vi "TrackerColor.vi"() -> ()   [LabVIEW 2015]
panel:
  in  "Example Image Path":path
  out "Image Out 2":T1(plugin-control)
  in  "Color":u32(colorbox)=16711680
  out "Image Out":T1(plugin-control)
  out "Image":T1(plugin-control)
  in  "Stop":bool
  out "Progress Bar":i32(slide) max=115 scale=1.0..115.0
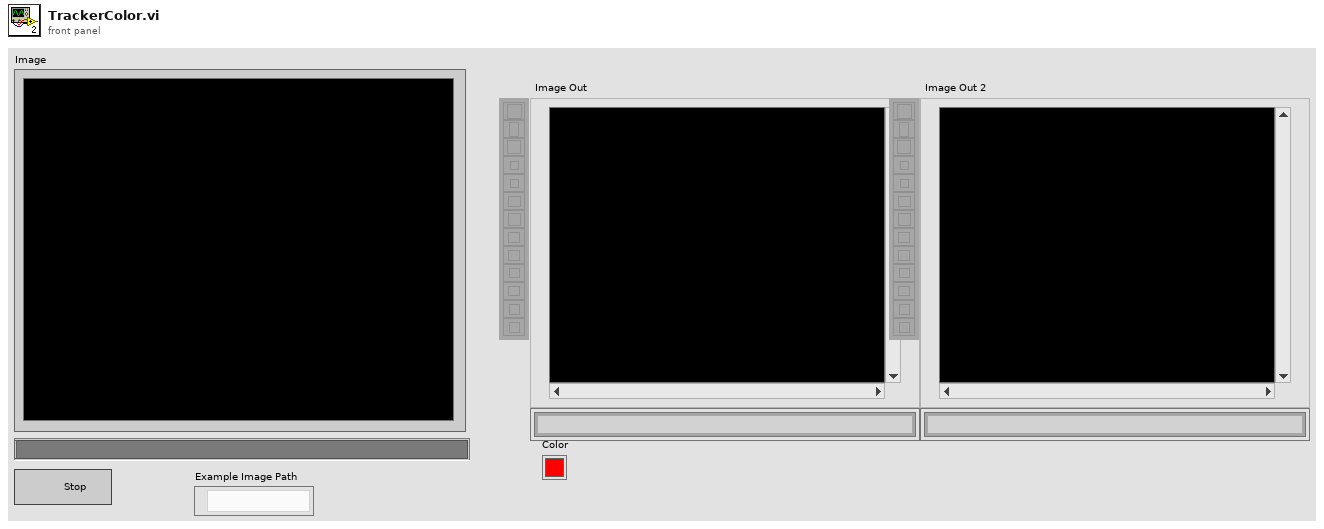
[diagram p1: front panel]
types:
  T1 = typedef "IMAQ Image.ctl" = refnum<image>
  T2 = typedef "IMAQ AVI2 Refnum.ctl" = refnum<k20>
  T3 = typedef "Image Type" = u32
  T4 = cluster{"Width":u32, "Height":u32, "Frames Per Second":u32, "Codec":string, "Has Data":bool}
  T5 = cluster{"Position":cluster{"x":sgl, "y":sgl}, "Angle":sgl, "Scale":sgl, "Score":sgl, "Bounding Box":cluster{"x":sgl, "y":sgl}[]}[]
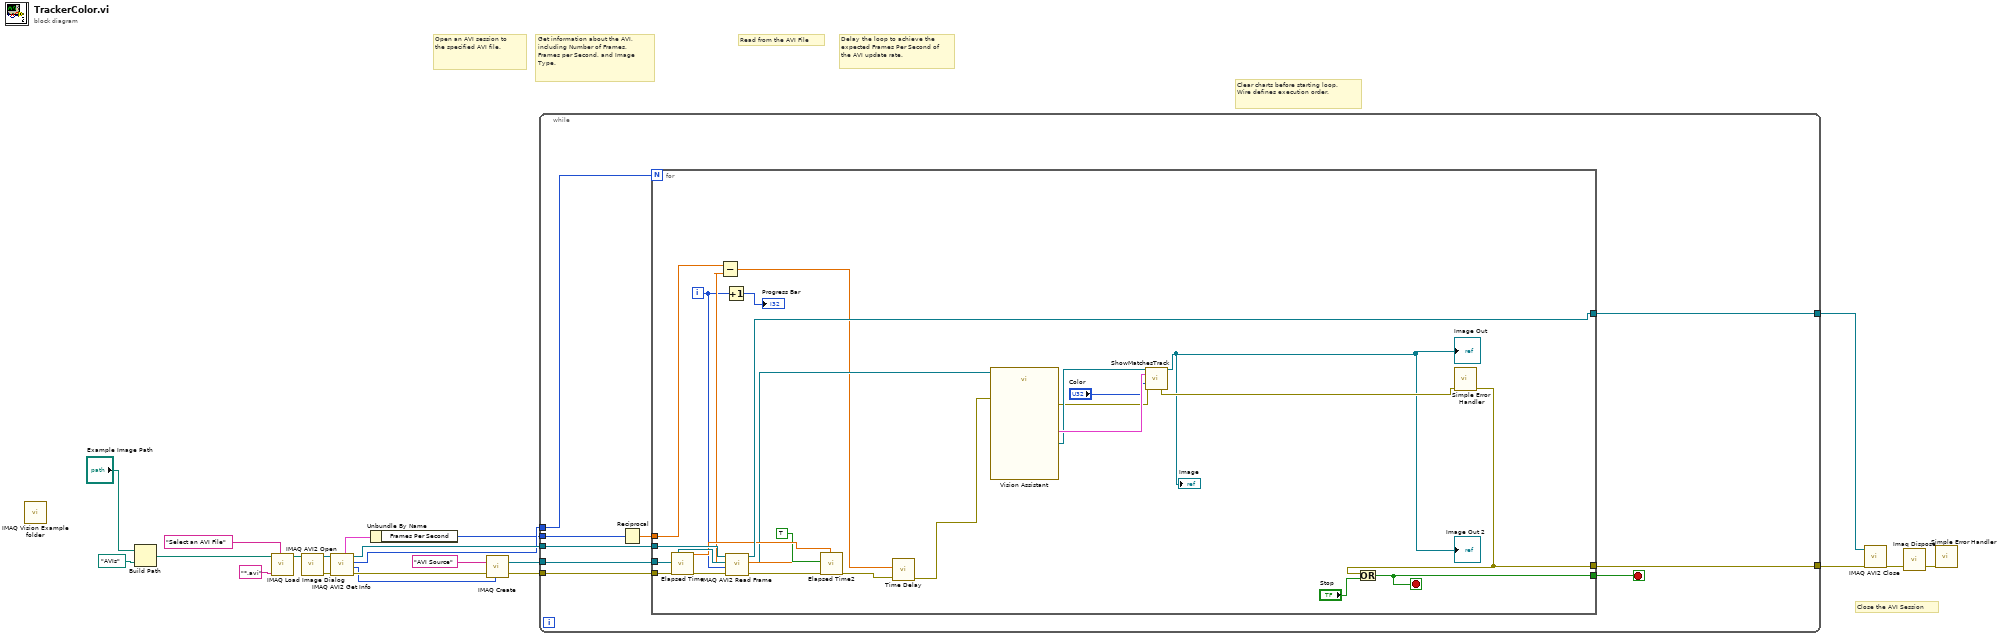
[diagram p0: block diagram]
diagram:
  # "Close the AVI Session"
  # "Clear charts before starting loop. Wire defines execution order."
  # "Read from the AVI File"
  # "Get information about the AVI, including Number of Frames, Frames per Second, and Image Type."
  # "Open an AVI session to the specified AVI file."
  # "Delay the loop to achieve the expected Frames Per Second of the AVI update rate."
  n1 = call "IMAQ Vision Example folder.vi"() -> ()  [unwired: 11 in, 1 out]
  n2 = Build Path(base path="Example Image Path", name or relative path=path "AVIs") -> (appended path=w6:path)
  n3 = call "IMAQ Load Image Dialog"("Prompt"="Select an AVI File" ("prompt"), "Pattern"="*.avi", "Start Path"=w6) -> ("Path"=w5:path)  [unwired: 6 in, 2 out]
  n4 = call "IMAQ AVI2 Open"("AVI File Path"=w5) -> ("error out"=w18:errorcluster, "AVI Refnum"=w17:T2)  [unwired: 2 in, 7 out]
  n5 = call "IMAQ AVI2 Get Info"("error in (no error)"=w18, "AVI Refnum"=w17) -> ("error out"=w14:errorcluster, "Image Type"=w9:T3, "Number of Frames"=w3:u32, "AVI Refnum (duplicate)"=w11:T2, "Frame Data"=w19:T4)  [unwired: 5 out]
  n6 = Unbundle By Name(w19) -> ("Frames Per Second"=w2:u32)
  n7 = call "IMAQ Create"("Image Name"="AVI Source", "Image Type"=w9, "error in (no error)"=w14) -> ("New Image"=w12:T1, "error out"=w13:errorcluster)  [unwired: 1 in, 1 out]
  n8 = while {
    tunnel: [w30] -> w16
    tunnel: [w29] -> w15
    tunnel: w13 -> [w28]
    tunnel: w12 -> [w27]
    tunnel: w11 -> [w26]
    tunnel: w2 -> [w25]
    tunnel: w3 -> [w23]
    stop <- w22 stop-if-true
    n9 = Reciprocal(x=w25) -> (1/x=w24:dbl)
    n10 = for {
      N: w23 -> [_]
      tunnel: w27 -> [w54]
      tunnel: [w53] -> w29
      tunnel: [w38] -> w30
      tunnel: w28 -> [w52]
      tunnel: w26 -> [w55]
      tunnel: w24 -> [w50]
      tunnel: [w40] -> w22
      i -> [w43]
      stop <- w40 stop-if-true
      n11 = call "Elapsed Time"("error in (no error)"=w52) -> ("Present (s)"=w49:dbl, "error out"=w51:errorcluster)  [unwired: 11 in, 6 out]
      n12 = Increment(x=w43) -> (x+1=→"Progress Bar":i32)
      n13 = call "IMAQ AVI2 Read Frame"("error in (no error)"=w51, "Frame Number"=w43, "Image"=w54, "AVI Refnum"=w55) -> ("error out"=w47:errorcluster, "Image Out"=w41:T1, "AVI Refnum (duplicate)"=w53:T2)  [unwired: 5 out]
      n14 = call "Elapsed Time2"("Reset"=TRUE, "error in (no error)"=w47, "Set Start Time (s)"=w49) -> ("Elapsed Time (s)"=w46:dbl, "error out"=w45:errorcluster)  [unwired: 9 in, 6 out]
      n15 = Subtract(x=w50, y=w46) -> (x-y=w32:dbl)
      n16 = call "Time Delay"("error in (no error)"=w45, "Delay Time (s)"=w32) -> ("error out"=w39:errorcluster)  [unwired: 9 in]
      n17 = call "Vision Assistant"("Image In"=w41, "error in"=w39) -> ("Image Out"=w36:T1, "Matches (Color Location 1)"=w37:T5, "error out"=w34:errorcluster)  [unwired: 21 in, 2 out]
      n18 = call "ShowMatchesTrack.vi"("Refnum in"=w36, "Matches (Color Location 3)"=w37, "Color"="Color", "error in (no error)"=w34) -> ("Refnum out"=→"Image" →"Image Out" →"Image Out 2":T1, "error out"=w33:errorcluster)  [unwired: 6 in, 4 out]
      n19 = call <vilib>:"Simple Error Handler.vi"("error in (no error)"=w33) -> ("error out"=w38:errorcluster)  [unwired: 1 in, 7 out]
      n20 = Or(x=w38, y="Stop") -> (x .or. y?=w40:bool)
    }
  }
  n21 = call "IMAQ AVI2 Close"("error in (no error)"=w16, "AVI Refnum"=w15) -> ("error out"=w10:errorcluster)  [unwired: 9 out]
  n22 = call "Imaq Dispose"("error in (no error)"=w10) -> ("error out"=w20:errorcluster)  [unwired: 2 in, 3 out]
  n23 = call <vilib>:"Simple Error Handler.vi"("error in (no error)"=w20) -> ()  [unwired: 1 in, 8 out]
